vi "Initialise UDP Link.vi"(9 "Port Number":u16, 10 "IP Address":string) -> (3 "UDP Link out":refnum<class "UDP Link.lvclass">)   [LabVIEW 2016, in "Assert API Components.lvlib" / "Assert Service.lvlib" / "UDP Link.lvlib" / "UDP Link.lvclass"]
uses:
  UDP Link.lvclass
  UDP Link.lvclass/UDP Link.ctl
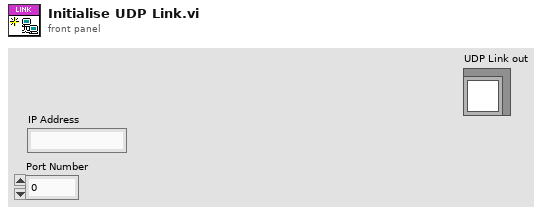
[diagram p1: front panel]
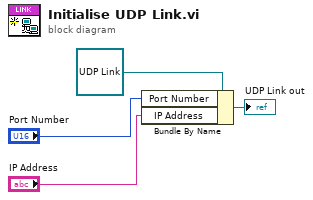
[diagram p0: block diagram]
diagram:
  n1 = Bundle By Name(cluster=refnum<class "UDP Link.lvclass"> refnum ("UDP Link in"), "Port Number"="Port Number", "IP Address"="IP Address") -> (→"UDP Link out":refnum<class "UDP Link.lvclass">)
